vi "constructor.vi"(8 "error in (no error)":errorcluster, 9 "remote port":u16, 10 "remote address":string, 11 "camera":string) -> (0 "error out":errorcluster, 3 "CameraNetworkController out":refnum<class "CameraNetworkController.lvclass">)   [LabVIEW 2011, in "Hardware.lvlib" / "HWControllers.lvlib" / "CameraNetworkController.lvclass"]
uses:
  CameraNetworkController.lvclass
  CameraNetworkController.lvclass/CameraNetworkController.ctl
  Channels/Camera/Camera/Camera.lvclass
  NetworkClient/NetworkServer.lvclass
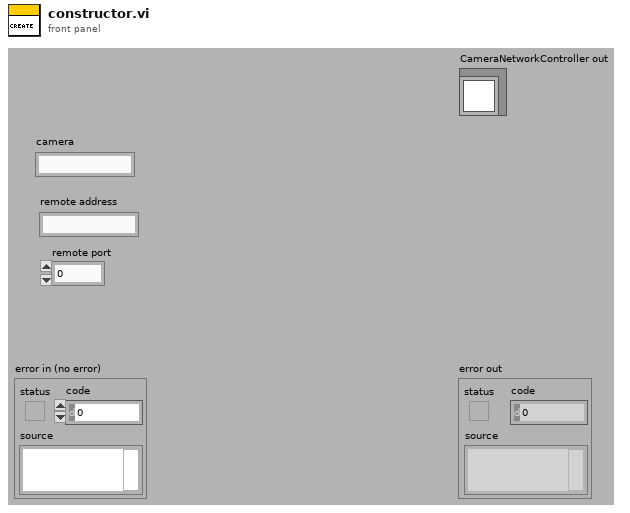
[diagram p1: front panel]
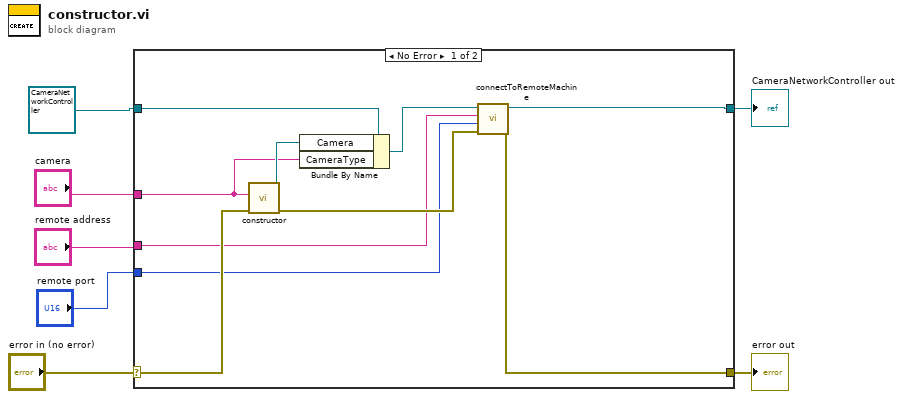
[diagram p0: block diagram]
diagram:
  n1 = case shown="No Error" "error in (no error)" {
    selector: "error in (no error)" -> [w17 w19]
    tunnel: [w11 w19] -> w6
    tunnel: [w12 w18] -> w5
    tunnel: refnum<class "CameraNetworkController.lvclass"> refnum ("Hardware:HWControllers.lvlib:CameraNetworkController.lvclass") -> [w16 w18]
    tunnel: "camera" -> [w14 _]
    tunnel: "remote address" -> [w9 _]
    tunnel: "remote port" -> [w8 _]
    frame No Error {
      n2 = call "constructor.vi"("error in (no error)"=w17, "Camera"=w14) -> ("error out"=w10:errorcluster, "Camera out"=w15:refnum<class "Camera.lvclass">)  [unwired: 8 in]
      n3 = Bundle By Name(cluster=w16, "Camera"=w15, "CameraType"=w14) -> (w13:refnum<class "CameraNetworkController.lvclass">)
      n4 = call "connectToRemoteMachine.vi"("error in (no error)"=w10, "remote port"=w8, "remote address"=w9, "NetworkServer in"=w13) -> ("error out"=w11:errorcluster, "NetworkServer out"=w12:refnum<class "CameraNetworkController.lvclass">)  [unwired: 6 in]
    }
    frame Error {
    }
  }
  "error out" <- w6
  "CameraNetworkController out" <- w5
